vi "Power Supply Change.vi"(6 "Priority Message? (F)":bool, 8 "error in":errorcluster, 11 "Power status":enum16{"OFF", "ON"}(ring)) -> (0 "error out":errorcluster)   [LabVIEW 2016]
uses:
  Message Queue/Message Queue.lvlib
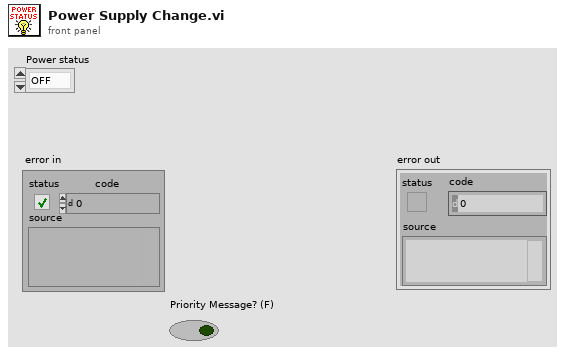
[diagram p1: front panel]
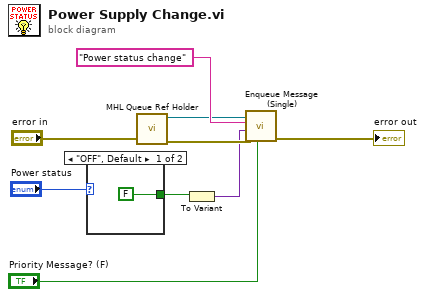
[diagram p0: block diagram]
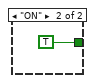
[diagram p2: hidden frame]
diagram:
  n1 = case shown="\"OFF\", Default" "Power status" {
    tunnel: [FALSE TRUE] -> w1
    frame "OFF", Default {
    }
    frame "ON" {
    }
  }
  n2 = call "MHL Queue Ref Holder.vi"("error in"="error in") -> ("error out"=w5:errorcluster, "Input Message Queue"=w6:refnum<queue>)  [unwired: 9 in]
  n3 = To Variant(anything=w1) -> (Variant=w4:variant)
  n4 = call "Enqueue Message (Single).vi"("Priority Message? (F)"="Priority Message? (F)", "error in (no error)"=w5, "Message Data"=w4, "Message"="Power status change", "Message Queue"=w6) -> ("error out"=→"error out":errorcluster)  [unwired: 5 in, 1 out]
